vi "createSaveTxtUniqueName.vi"(8 "error in (no error)":errorcluster, 9 "save to":path) -> (0 "error out":errorcluster, 2 "refnum out":refnum<file>, 3 "actuall saving path":path=path "C:/temp/test_020.txt")   [LabVIEW 2021]
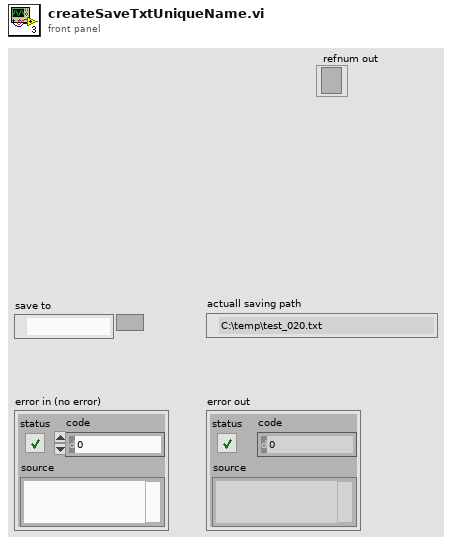
[diagram p1: front panel]
types:
  T1 = enum16{"open", "replace", "create", "open or create", "replace or create", "replace or create with confirmation"}
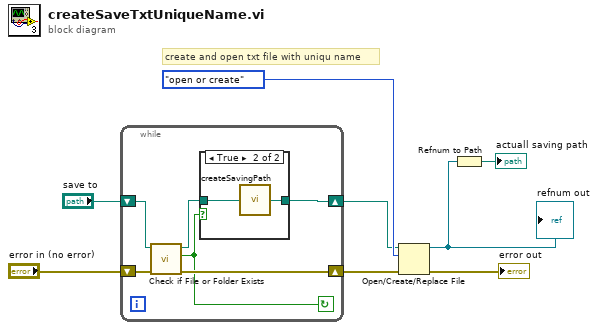
[diagram p0: block diagram]
diagram:
  # "create and open txt file with uniqu name"
  n1 = while {
    shift-right: [w14] -> w6
    shift-left: "save to" -> [w12]
    shift-right: [w13] -> w5
    shift-left: "error in (no error)" -> [w11]
    stop <- w9 continue-if-true
    n2 = call <vilib>:"Check if File or Folder Exists.vi"("error in (no error)"=w11, "path"=w12) -> ("error out"=w13:errorcluster, "file or folder exists?"=w9:bool, "dup path"=w10:path)  [unwired: 7 in]
    n3 = case shown="True" w9 {
      tunnel: w10 -> [w15 w17]
      tunnel: [w15 w16] -> w14
      frame False {
      }
      frame True {
        n4 = call "createSavingPath.vi"("pathIn"=w17) -> ("pathOut"=w16:path)
      }
    }
  }
  n5 = Open/Create/Replace File(file path (use dialog)=w6, error in=w5, operation (0:open)=T1."open or create") -> (refnum out=w1:refnum<file>, error out=→"error out":errorcluster)  [unwired: 3 in, 1 out]
  "refnum out" <- w1
  n6 = Refnum to Path(1:w1) -> (0:→"actuall saving path":path)
